vi "Actor Core.vi"(8 "error in":errorcluster, 11 "Measure Object in":refnum<class "Log Record.lvclass">) -> (0 "error out":errorcluster, 3 "Actor out":refnum<class "Actor.lvclass">)   [LabVIEW 2024, in "Log Record.lvclass"]
doc: "(<B>Filename</B>: Actor Framework.lvlib:Actor.lvclass:Actor Core.vi)\n\nReceives messages to the actor, reacts to them, and initiates any error handling that may shut the actor down.\n\nDescendant classes may override this VI to append parallel tasks for the actor to complete while it handles messages. Overrides use the Call Parent Method node."
uses:
  Log Record.lvclass
  C:/Git/LabActor/Template Module/Template Module.lvclass
  C:/Program Files/National Instruments/LabVIEW 2024/vi.lib/ActorFramework/Actor/Actor.lvclass
  <vilib>/ActorFramework/Actor/Actor.lvclass
  Log Record Configuration.ctl
  NHMFL_Core/Libraries/FAIR Data/MagX/Add-on Storage.ctl
  Log Record.lvclass/Log Record.ctl
  Template Module/Template Module.lvclass/Template Module.ctl
  <vilib>/ActorFramework/Actor/Actor.lvclass/Actor.ctl
  <vilib>/ActorFramework/Message Enqueuer/Message Enqueuer.lvclass/Message Enqueuer.ctl
  Log Record Messages/Set Metadata Msg/Set Metadata Msg.lvclass/Set Metadata Msg.ctl
  Log Record Messages/Set Instruments Msg/Set Instruments Msg.lvclass/Set Instruments Msg.ctl
  Controllers/Application Controller Messages/Help Msg/Help Msg.lvclass/Help Msg.ctl
  Log Record Messages/Write Add-on storage Msg/Write Add-on storage Msg.lvclass/Write Add-on storage Msg.ctl
  Template Module/Read stop event.vi
  Template Module/Read Name.vi
  <vilib>/ActorFramework/Message Enqueuer/Init from Existing Queue.vi
  <vilib>/ActorFramework/Message Enqueuer/Enqueue.vi
  Log Record Messages/Set Metadata Msg/Set Metadata Msg.lvclass
  C:/Program Files/National Instruments/LabVIEW 2024/vi.lib/ActorFramework/Message/Message.lvclass
  Log Record Messages/Set Instruments Msg/Set Instruments Msg.lvclass
  Controllers/Application Controller Messages/Help Msg/Help Msg.lvclass
  Log Record Messages/Write Add-on storage Msg/Write Add-on storage Msg.lvclass
  Log Record Messages/OSF Sync Command Msg/OSF Sync Command Msg.lvclass
  <vilib>/ActorFramework/Message Priority Queue/Priority Enqueue.vi
  <vilib>/Platform/browser.llb/Open URL in Default Browser (string).vi
  Process Object/Process Object.lvclass
  <vilib>/ActorFramework/Message Enqueuer/Message Enqueuer.lvclass
panel:
  out "Online":bool
  in  "Help Button":bool
  out "Principal Investigator":string
  out "Probe":string
  in  "Storage location":T1=enum."OSF - Split"
  out "Experiment":string
  out "OSF user":string
  in  "Logon":bool
  out "Experiment title":string
  in  "Change experiment":bool
  out "Project title":string
  in  "OSF Token":string
  in  "Configuration":T2={"OSF node  ID"="", "Conection timeout"=60.0, "Station"="Cell_1", "Log server "="magx.lanl.gov", "Upload to OSF"=FALSE, "Append to lab book"=FALSE, "Filing modules"=["Monitor Controller", "Pulse Controller", "LabActor", "File Converter"], "File prefix"="_c4_", "Computer"=""} {"Conection timeout" format="%#_6ps"}
  in  "Re-process":bool
  in  "Input file":path
  out "Name":string
  in  "Change probe":bool
  in  "View hub":bool
  # "OSF Syncronization"
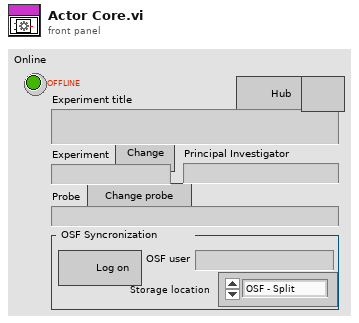
[diagram p1: front panel]
types:
  T1 = typedef "Add-on Storage.ctl" = enum16{"OSF", "OSF - Split", "Google Drive", "Dropbox", "Box"}
  T2 = typedef "Log Record Configuration.ctl" = cluster{"OSF node  ID":string, "Conection timeout":dbl, "Station":string, "Log server ":string, "Upload to OSF":bool, "Append to lab book":bool, "Filing modules":string[], "File prefix":string, "Computer":string}
  T3 = typedef "Experiment info.ctl" = cluster{"attendee":string[], "title":string, "magnet_System":string, "proposal_Number":string, "proposal_Title":string, "facility":string, "pi":string, "dtstart":string, "dtend":string, "dtstamp":string, "location":string, "summary":string, "pid":string, "support":string, "uid":string, "start":u64, "id":u64}
  T4 = typedef "Instrument info.ctl" = cluster{"instrumentPid":string, "title":string, "filename":string, "filestorePath":string, "createDate":string, "modifyDate":string, "categories":string, "instrumenType":string}
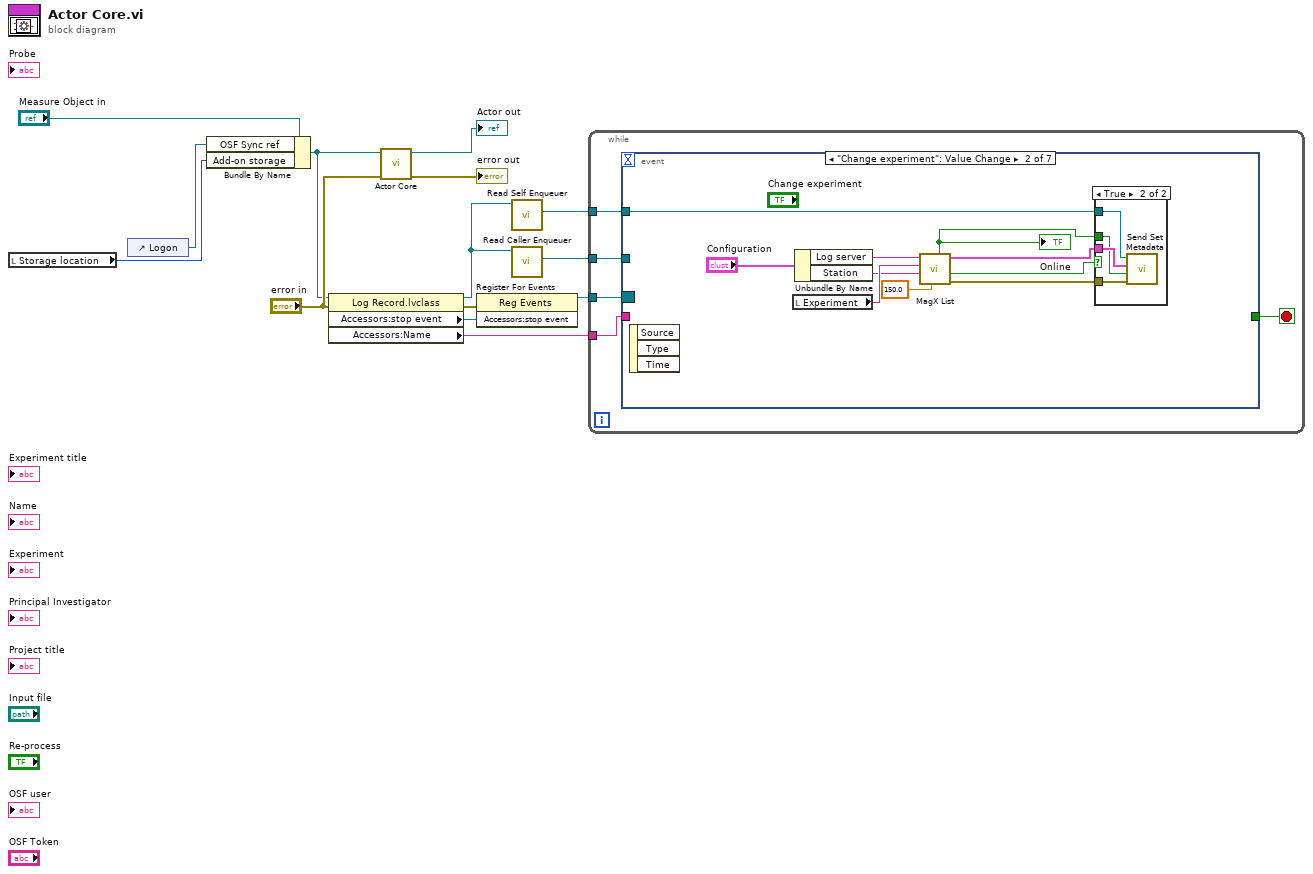
[diagram p0: block diagram]
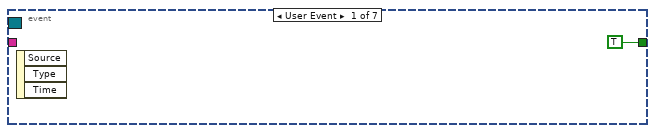
[diagram p2: hidden frame]
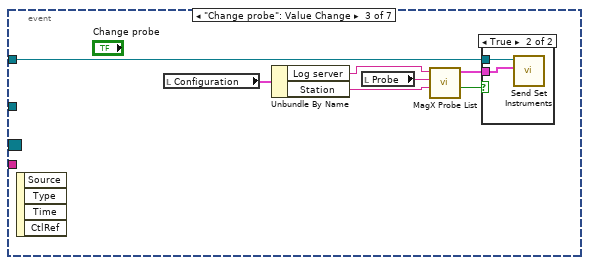
[diagram p4: hidden frame]
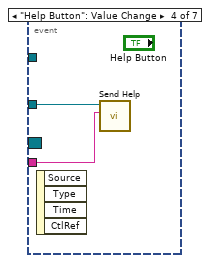
[diagram p6: hidden frame]
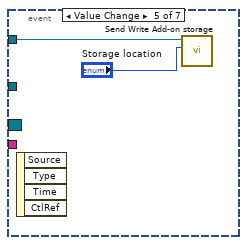
[diagram p7: hidden frame]
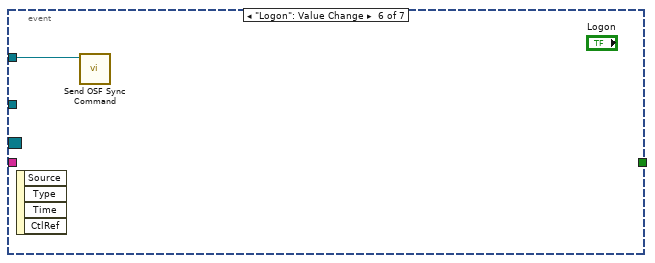
[diagram p8: hidden frame]
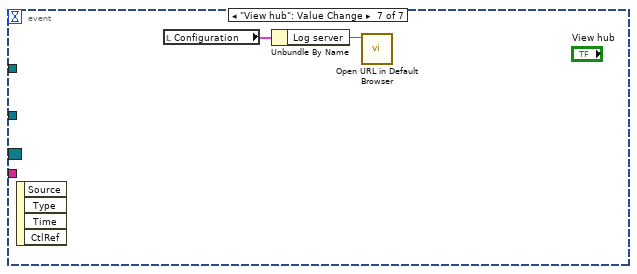
[diagram p9: hidden frame]
diagram:
  n1 = local read "Storage location"() -> (w4:T1)
  n2 = control-ref of="Logon"() -> (w5:refnum<vi>)
  n3 = Bundle By Name(cluster="Measure Object in", "OSF Sync ref"=w5, "Add-on storage"=w4) -> (w6:refnum<class "Log Record.lvclass">)
  n4 = property class="Log Record.lvclass"(reference=w6, error in="error in") -> (reference out=w3:refnum<class "Log Record.lvclass">, error out=w12:errorcluster, "Accessors:stop event"=w11:refnum<user-event>, "Accessors:Name"=w1:string)
  n5 = call-parent "Actor Core.vi"("error in"="error in", "Measure Object in"=w6) -> ("error out"=→"error out":errorcluster, "Actor out"=→"Actor out":refnum<class "Actor.lvclass">)  [unwired: 8 in]
  n6 = register-events(error in=w12, w11) -> (reference out=w10:refnum<event-registration>)  [unwired: 1 in, 1 out]
  n7 = call <vilib>:"Read Self Enqueuer.vi"("Actor"=w3) -> ("Self Enqueuer"=w7:refnum<class "Message Enqueuer.lvclass">)  [unwired: 10 in]
  n8 = call <vilib>:"Read Caller Enqueuer.vi"("Actor"=w3) -> ("Caller Enqueuer"=w2:refnum<class "Message Enqueuer.lvclass">)  [unwired: 10 in]
  n9 = while {
    tunnel: w10 -> [w19]
    tunnel: w7 -> [w17]
    tunnel: w2 -> [w16]
    tunnel: w1 -> [w15]
    stop <- w18 stop-if-true
    n10 = event shown="[1] \"Change experiment\": Value Change" {
      selector: w19 -> [_ _ _ _ _ _ _]
      dyn-events: _ -> [_ _ _ _ _ _ _]
      timeout: _ -> [_ _ _ _ _ _ _]
      tunnel: [TRUE _ _ _ _ _ _] -> w18
      tunnel: w17 -> [_ w29 w36 _ w47 w48 _]
      tunnel: w16 -> [_ _ _ w45 _ _ _]
      tunnel: w15 -> [_ _ _ w44 _ _ _]
      event User Event {
        n11 = event-data() -> ()  [unwired: 1 in, 3 out]
      }
      event "Change experiment": Value Change {
        n12 = event-data() -> ()  [unwired: 1 in, 3 out]
        n13 = local read "Experiment"() -> (w30:string)
        n14 = Unbundle By Name("Configuration") -> ("Log server"=w22:string, "Station"=w23:string)
        n15 = call "MagX List.vi"("Days range"=150.0, "Current station in"=w23, "Initial Selection"=w30, "Hub URL"=w22) -> ("error out"=w26:errorcluster, "OK"=w28:bool, "Experiment info"=w27:T3, "Online"=w21:bool)  [unwired: 4 in]
        "Online" <- w21
        n16 = case shown="True" w28 {
          tunnel: w29 -> [_ w34]
          tunnel: w27 -> [_ w33]
          tunnel: w26 -> [_ w32]
          tunnel: w21 -> [_ w31]
          frame False {
          }
          frame True {
            n17 = call "Send Set Metadata.vi"("error in (no error)"=w32, "Online"=w31, "Experiment info"=w33, "Message Enqueuer"=w34) -> ()  [unwired: 6 in, 2 out]
          }
        }
      }
      event "Change probe": Value Change {
        n18 = event-data() -> ()  [unwired: 1 in, 4 out]
        n19 = local read "Configuration"() -> (w41:T2)
        n20 = Unbundle By Name(w41) -> ("Log server"=w40:string, "Station"=w39:string)
        n21 = local read "Probe"() -> (w38:string)
        n22 = call "MagX Probe List.vi"("Current station in"=w39, "Initial Selection"=w38, "Hub URL"=w40) -> ("OK"=w37:bool, "Probe info"=w35:T4)  [unwired: 6 in, 1 out]
        n23 = case shown="True" w37 {
          tunnel: w36 -> [_ w43]
          tunnel: w35 -> [_ w42]
          frame False {
          }
          frame True {
            n24 = call "Send Set Instruments.vi"("Instrument info"=w42, "Message Enqueuer"=w43) -> ()  [unwired: 8 in, 2 out]
          }
        }
      }
      event "Help Button": Value Change {
        n25 = event-data() -> ()  [unwired: 1 in, 4 out]
        n26 = call "Send Help.vi"("Module name"=w44, "Message Enqueuer"=w45) -> ()  [unwired: 8 in, 2 out]
      }
      event Value Change {
        n27 = event-data() -> ()  [unwired: 1 in, 4 out]
        n28 = call "Send Write Add-on storage.vi"("Add-on storage"="Storage location", "Message Enqueuer"=w47) -> ()  [unwired: 8 in, 2 out]
      }
      event "Logon": Value Change {
        n29 = event-data() -> ()  [unwired: 1 in, 4 out]
        n30 = call "Send OSF Sync Command.vi"("Message Enqueuer"=w48) -> ()  [unwired: 9 in, 2 out]
      }
      event "View hub": Value Change {
        n31 = event-data() -> ()  [unwired: 1 in, 4 out]
        n32 = local read "Configuration"() -> (w50:T2)
        n33 = Unbundle By Name(w50) -> ("Log server"=w49:string)
        n34 = call-poly <vilib>:"Open URL in Default Browser.vi"("URL"=w49) -> ()  [unwired: 5 in, 2 out]
      }
    }
  }
